vi "SP Initialize Test.vi"(0 "Instrument Record":T9, 2 "Files Found?":bool=TRUE, 5 "Parent VI Refnum":refnum<vi>, 7 "Timing Metrics In":string, 9 "Test Parameters":T10={"Stimulus"={"Use Instrument Settings"=FALSE, "Blank Frequencies"=FALSE, "Sweep Type"=enum."Linear", "Sweep"={"Fstart"=500.0, "Fstop"=1500.0, "Units"=enum."MHz", "Points"=2}, "Power (dBm)"=999.0, "IFBW (Hz)"=-1.0, "Sweep Time (s)"=-1.0, "Calibration"={"State"=FALSE, "String"=""}}, "Measurement"={"Auto Select"=TRUE, "Data Source"=enum."VNA", "Ports"=2, "Parameters"=[]}, "De-Embed"={"De-Embed"=FALSE, "Adapters"=[]}, "Display"={"Lock Control"=FALSE, "Retain Settings"=TRUE, "Formatted Data"=FALSE, "Plot Orientation"=enum."Single", "Plot Controls"=[{"Trace Orientation"=enum."Overlay", "Frequency"={"Change Frequency"=FALSE, "Start"=500.0, "Stop"=1500.0, "Units"=enum."MHz"}, "Markers"=[], "Traces"=[]}, {"Trace Orientation"=enum."Overlay", "Frequency"={"Change Frequency"=FALSE, "Start"=500.0, "Stop"=1500.0, "Units"=enum."MHz"}, "Markers"=[], "Traces"=[]}, {"Trace Orientation"=enum."Overlay", "Frequency"={"Change Frequency"=FALSE, "Start"=500.0, "Stop"=1500.0, "Units"=enum."MHz"}, "Markers"=[], "Traces"=[]}, {"Trace Orientation"=enum."Overlay", "Frequency"={"Change Frequency"=FALSE, "Start"=500.0, "Stop"=1500.0, "Units"=enum."MHz"}, "Markers"=[], "Traces"=[]}]}, "Limits"=[], "Filter Limits"=[]} {"Filter Limits"."Parameter"."Stimulus Port" min=1 step=1; "Filter Limits"."Parameter"."Response Port" min=1 step=1; "Filter Limits"."Passband"."Bandwidth Attn" format="%.3g"; "Filter Limits"."Passband"."Stop/Span" format="%.3g"; "Filter Limits"."Passband"."Start/Center" format="%.3g"; "Measurement"."Parameters"."Channel" min=0 max=32 step=1; "Measurement"."Parameters"."Parameter"."Stimulus Port" min=1 step=1; "Measurement"."Parameters"."Parameter"."Response Port" min=1 step=1; "Limits"."Parameter"."Stimulus Port" min=1 step=1; "Limits"."Parameter"."Response Port" min=1 step=1; "Stimulus"."Sweep Time (s)" format="%.3g"; "Display"."Plot Controls"."Traces"."Reference" format="%#.2g"; "Display"."Plot Controls"."Traces"."Display Data" items=["Data", "Memory", "Data/Memory"]; "Display"."Plot Controls"."Traces"."Format" items=["Log Mag", "Phase", "Expanded Phase", "Delay", "Smith", "Polar", "Lin Mag", "SWR", "Loss", "Real", "Imaginary"]; "Display"."Plot Controls"."Traces"."Scale" min=0.001 step=1.0 format="%#.2g"; "Display"."Plot Controls"."Traces"."Position" min=0.0 max=10.0; "Display"."Plot Controls"."Frequency"."Stop" format="%.3g"; "Display"."Plot Controls"."Frequency"."Start" format="%.3g"}, 11 "error in (no error)":errorcluster, 12 "Seq Count":u32) -> (4 "Instrument ID":string, 6 "Next Action":string, 8 "Timing Metrics Out":string, 10 "dup Test Parameters":T10={"Stimulus"={"Use Instrument Settings"=FALSE, "Blank Frequencies"=FALSE, "Sweep Type"=enum."Linear", "Sweep"={"Fstart"=500.0, "Fstop"=1500.0, "Units"=enum."MHz", "Points"=2}, "Power (dBm)"=999.0, "IFBW (Hz)"=-1.0, "Sweep Time (s)"=-1.0, "Calibration"={"State"=FALSE, "String"=""}}, "Measurement"={"Auto Select"=TRUE, "Data Source"=enum."VNA", "Ports"=2, "Parameters"=[]}, "De-Embed"={"De-Embed"=FALSE, "Adapters"=[]}, "Display"={"Lock Control"=FALSE, "Retain Settings"=TRUE, "Formatted Data"=FALSE, "Plot Orientation"=enum."Single", "Plot Controls"=[{"Trace Orientation"=enum."Overlay", "Frequency"={"Change Frequency"=FALSE, "Start"=500.0, "Stop"=1500.0, "Units"=enum."MHz"}, "Markers"=[], "Traces"=[]}, {"Trace Orientation"=enum."Overlay", "Frequency"={"Change Frequency"=FALSE, "Start"=500.0, "Stop"=1500.0, "Units"=enum."MHz"}, "Markers"=[], "Traces"=[]}, {"Trace Orientation"=enum."Overlay", "Frequency"={"Change Frequency"=FALSE, "Start"=500.0, "Stop"=1500.0, "Units"=enum."MHz"}, "Markers"=[], "Traces"=[]}, {"Trace Orientation"=enum."Overlay", "Frequency"={"Change Frequency"=FALSE, "Start"=500.0, "Stop"=1500.0, "Units"=enum."MHz"}, "Markers"=[], "Traces"=[]}]}, "Limits"=[], "Filter Limits"=[]} {"Filter Limits"."Parameter"."Stimulus Port" min=1 step=1; "Filter Limits"."Parameter"."Response Port" min=1 step=1; "Filter Limits"."Passband"."Bandwidth Attn" format="%.3g"; "Filter Limits"."Passband"."Stop/Span" format="%.3g"; "Filter Limits"."Passband"."Start/Center" format="%.3g"; "Measurement"."Parameters"."Channel" min=0 max=32 step=1; "Measurement"."Parameters"."Parameter"."Stimulus Port" min=1 step=1; "Measurement"."Parameters"."Parameter"."Response Port" min=1 step=1; "Limits"."Parameter"."Stimulus Port" min=1 step=1; "Limits"."Parameter"."Response Port" min=1 step=1; "Stimulus"."Sweep Time (s)" format="%.3g"; "Display"."Plot Controls"."Traces"."Reference" format="%#.2g"; "Display"."Plot Controls"."Traces"."Display Data" items=["Data", "Memory", "Data/Memory"]; "Display"."Plot Controls"."Traces"."Format" items=["Log Mag", "Phase", "Expanded Phase", "Delay", "Smith", "Polar", "Lin Mag", "SWR", "Loss", "Real", "Imaginary"]; "Display"."Plot Controls"."Traces"."Scale" min=0.001 step=1.0 format="%#.2g"; "Display"."Plot Controls"."Traces"."Position" min=0.0 max=10.0; "Display"."Plot Controls"."Frequency"."Stop" format="%.3g"; "Display"."Plot Controls"."Frequency"."Start" format="%.3g"}, 14 "Driver Ref":T5, 15 "error out":errorcluster {"code" format="%.0x"})   [LabVIEW 2011]
uses:
  TypeDefs/SP Test Parameters.ctl
  TypeDefs/SP Stimulus Parameters.ctl
  TypeDefs/SP Frequency Units.ctl
  TypeDefs/SP Calibration State.ctl
  TypeDefs/SP Measurement.ctl
  TypeDefs/SP Parameters.ctl
  TypeDefs/SP Parameter.ctl
  TypeDefs/SP De-Embed.ctl
  TypeDefs/SP Adapter.ctl
  TypeDefs/SP Data.ctl
  TypeDefs/SP Display Parameters.ctl
  TypeDefs/SP Display Plot Controls Cluster.ctl
  TypeDefs/SP Marker Cluster.ctl
  TypeDefs/SP Marker Type.ctl
  TypeDefs/SP Display Trace Controls.ctl
  TypeDefs/SP Display Format.ctl
  TypeDefs/SP Display Data.ctl
  TypeDefs/SP Limit.ctl
  TypeDefs/SP Format.ctl
  TypeDefs/SP Limit Type.ctl
  TypeDefs/SP Limit Point.ctl
  Test Referential Limit.ctl
  TypeDefs/SP Filter.ctl
  TypeDefs/SP Filter Type.ctl
  TypeDefs/SP Filter Passband.ctl
  TypeDefs/SP Frequency Format.ctl
  TypeDefs/SP Filter Ripple.ctl
  TypeDefs/SP Attenuation Point.ctl
  TypeDefs/SP Attenuation Type.ctl
  TypeDefs/SP Skirt Rejection Point.ctl
  TypeDefs/SP Relative Loss.ctl
  typedefs/Instrument Record.ctl
  TypeDefs/SP Driver Refs.ctl
  drivers/VNA/VNA Driver Ref.ctl
  drivers/SNA/SNA Driver Ref.ctl
  drivers/IMP/IMP Driver Ref.ctl
  TypeDefs/SP Parameter to Measure.ctl
  TypeDefs/SP Measurement Format.ctl
  TypeDefs/SP Miscellaneous Parameters.ctl
  drivers/VNA/VNA Command.ctl
  drivers/SNA/SNA Command.ctl
  drivers/IMP/IMP Command.ctl
panel:
  out "Parameters to Measure":T1[](array[typedef]) {"Channel" min=1 max=99 step=1; "Parameter"."Stimulus Port" min=1 step=1; "Parameter"."Response Port" min=1 step=1}
  # "Div"
  # "Div"
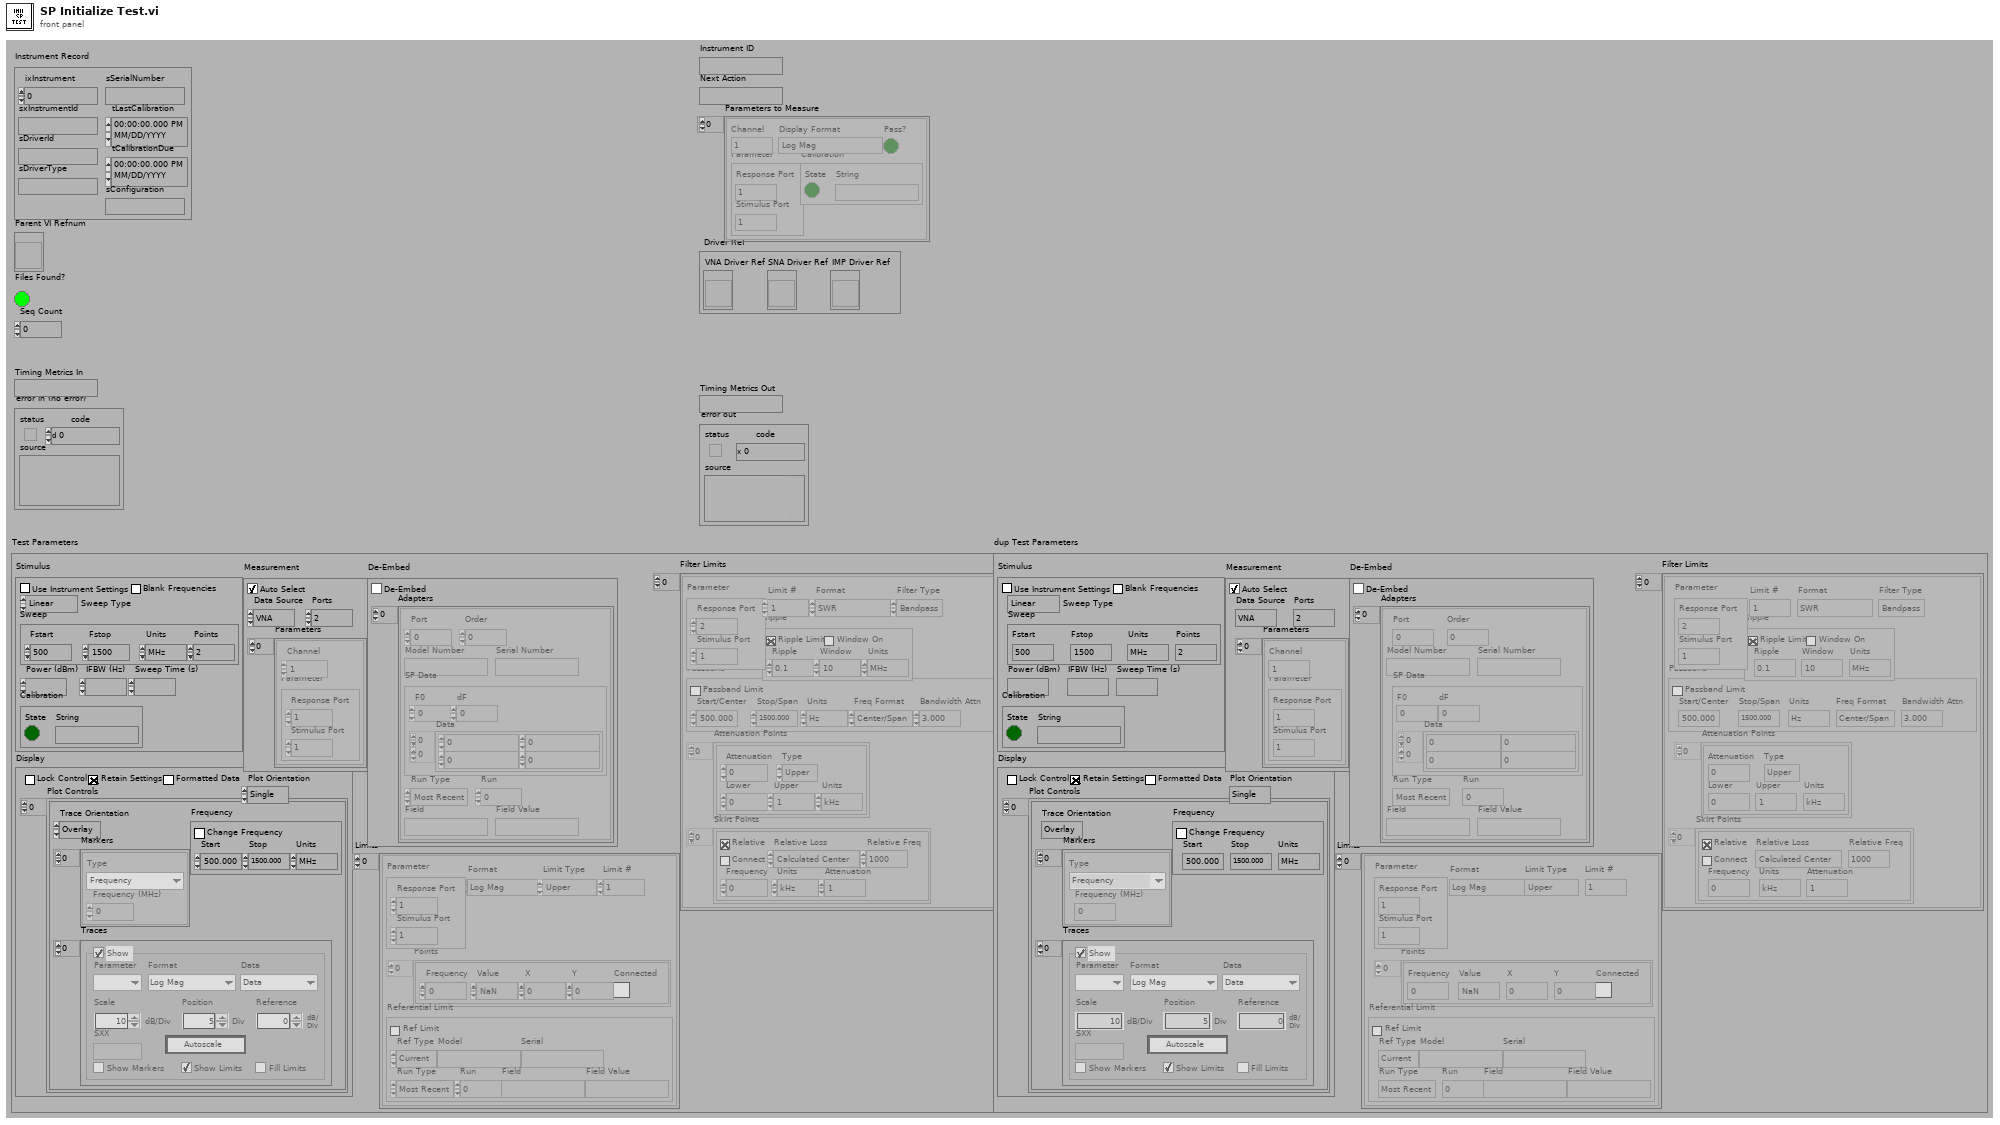
[diagram p1: front panel]
types:
  T1 = typedef "SP Parameter to Measure.ctl" = cluster{"Channel":i8, "Parameter":T2, "Calibration":T3, "Display Format":T4, "Pass?":bool}
  T2 = typedef "SP Parameter.ctl" = cluster{"Stimulus Port":i8, "Response Port":i8}
  T3 = typedef "SP Calibration State.ctl" = cluster{"State":bool, "String":string}
  T4 = typedef "SP Measurement Format.ctl" = enum32{"Log Mag", "Phase", "Delay", "Smith (R+jX)", "Polar (Re/Im)", "Linear Mag", "SWR", "Real", "Imaginary", "Smith (Lin/Phase)", "Smith (Log/Phase)", "Smith (Real/Imag)", "Smith (G+jB)", "Polar (Lin/Phase)", "Polar (Log/Phase)", "Expanded Phase", "Positive Phase", "Inverted Smith", "Unwrapped Phase", "Power Out", "Power In", "Linear Mag/Phase", "Log Mag/Phase", "Real/Imaginary"}
  T5 = typedef "SP Driver Refs.ctl" = cluster{"VNA Driver Ref":T6, "SNA Driver Ref":T7, "IMP Driver Ref":T8}
  T6 = typedef "VNA Driver Ref.ctl" = refnum<vi>
  T7 = typedef "SNA Driver Ref.ctl" = refnum<vi>
  T8 = typedef "IMP Driver Ref.ctl" = refnum<vi>
  T9 = typedef "Instrument Record.ctl" = cluster{"ixInstrument":i32, "sxInstrumentId":string, "sDriverId":string, "sDriverType":string, "sSerialNumber":string, "tLastCalibration":timestamp, "tCalibrationDue":timestamp, "sConfiguration":string}
  T10 = typedef "SP Test Parameters.ctl" = cluster{"Stimulus":T11, "Measurement":T13, "De-Embed":T15, "Display":T18, "Limits":T25[], "Filter Limits":T30[]}
  T11 = typedef "SP Stimulus Parameters.ctl" = cluster{"Use Instrument Settings":bool, "Blank Frequencies":bool, "Sweep Type":enum32{"Linear", "Logarithmic", "List", "Power", "CW"}, "Sweep":cluster{"Fstart":dbl, "Fstop":dbl, "Units":T12, "Points":i32}, "Power (dBm)":dbl, "IFBW (Hz)":dbl, "Sweep Time (s)":dbl, "Calibration":T3}
  T12 = typedef "SP Frequency Units.ctl" = enum16{"Hz", "kHz", "MHz", "GHz", "Points"}
  T13 = typedef "SP Measurement.ctl" = cluster{"Auto Select":bool, "Data Source":enum16{"VNA", "Data File"}, "Ports":i8, "Parameters":T14[]}
  T14 = typedef "SP Parameters.ctl" = cluster{"Channel":i8, "Parameter":T2}
  T15 = typedef "SP De-Embed.ctl" = cluster{"De-Embed":bool, "Adapters":T16[]}
  T16 = typedef "SP Adapter.ctl" = cluster{"Port":i8, "Order":i8, "Model Number":string, "Serial Number":string, "SP Data":T17, "Run Type":enum16{"Most Recent", "Run #", "Match Field"}, "Run":i32, "Field":string, "Field Value":string}
  T17 = typedef "SP Data.ctl" = cluster{"F0":dbl, "dF":dbl, "Data":cdb[][]}
  T18 = typedef "SP Display Parameters.ctl" = cluster{"Lock Control":bool, "Retain Settings":bool, "Formatted Data":bool, "Plot Orientation":enum32{"Single", "Dual", "Quad"}, "Plot Controls":T19[]}
  T19 = typedef "SP Display Plot Controls Cluster.ctl" = cluster{"Trace Orientation":enum32{"Overlay", "Split"}, "Frequency":cluster{"Change Frequency":bool, "Start":dbl, "Stop":dbl, "Units":T12}, "Markers":T20[], "Traces":T22[]}
  T20 = typedef "SP Marker Cluster.ctl" = cluster{"Type":T21, "Frequency (MHz)":dbl}
  T21 = typedef "SP Marker Type.ctl" = enum16{"Frequency", "Trace Maximum", "Trace Minimum", "Limit Maximum", "Limit Minimum"}
  T22 = typedef "SP Display Trace Controls.ctl" = cluster{"Trace On":bool, "Measure":i32, "Format":T23, "Autoscale":bool, "Reference":dbl, "\nRefUnit":string, "Position":dbl, "Scale":dbl, "ScaleUnit":string, "LimitOn":bool, "LimitFill":bool, "Display Data":T24, "Show Markers":bool, "SXX":string}
  T23 = typedef "SP Display Format.ctl" = i32
  T24 = typedef "SP Display Data.ctl" = u16
  T25 = typedef "SP Limit.ctl" = cluster{"Parameter":T2, "Format":T26, "Limit Type":T27, "Points":T28[], "Referential Limit":T29, "Limit #":i8}
  T26 = typedef "SP Format.ctl" = enum16{"Log Mag", "Lin Mag", "SWR", "Phase", "Expanded Phase", "Delay", "Insertion Loss", "Isolation", "Return Loss"}
  T27 = typedef "SP Limit Type.ctl" = enum16{"Upper", "Lower", "Delta", "Filter", "Referential"}
  T28 = typedef "SP Limit Point.ctl" = cluster{"Frequency":dbl, "Value":dbl, "X":dbl, "Y":dbl, "Connected":bool}
  T29 = typedef "Test Referential Limit.ctl" = cluster{"Ref Limit":bool, "Ref Type":enum16{"Current", "Specify"}, "Model":string, "Serial":string, "Run Type":enum16{"Most Recent", "Run #", "Match Field"}, "Run":i32, "Field":string, "Field Value":string}
  T30 = typedef "SP Filter.ctl" = cluster{"Limit #":i8, "Parameter":T2, "Format":T26, "Filter Type":T31, "Passband":T32, "Ripple":T34, "Attenuation Points":T35[], "Skirt Points":T37[]}
  T31 = typedef "SP Filter Type.ctl" = enum16{"Lowpass", "Highpass", "Bandpass", "Bandstop"}
  T32 = typedef "SP Filter Passband.ctl" = cluster{"Start/Center":dbl, "Stop/Span":dbl, "Units":T12, "Freq Format":T33, "Bandwidth Attn":dbl, "Passband Limit":bool}
  T33 = typedef "SP Frequency Format.ctl" = enum16{"Start/Stop", "Center/Span"}
  T34 = typedef "SP Filter Ripple.ctl" = cluster{"Ripple Limit":bool, "Window On":bool, "Ripple":dbl, "Window":dbl, "Units":T12}
  T35 = typedef "SP Attenuation Point.ctl" = cluster{"Attenuation":dbl, "Type":T36, "Lower":dbl, "Upper":dbl, "Units":T12}
  T36 = typedef "SP Attenuation Type.ctl" = enum16{"Center", "Lower", "Upper"}
  T37 = typedef "SP Skirt Rejection Point.ctl" = cluster{"Relative":bool, "Connect":bool, "Frequency":dbl, "Units":T12, "Attenuation":dbl, "Relative Loss":T38, "Relative Freq":dbl}
  T38 = typedef "SP Relative Loss.ctl" = enum16{"Calculated Center", "Passband Minimum", "Passband Maximum", "Passband Average", "Frequency"}
  T39 = typedef "SP Miscellaneous Parameters.ctl" = cluster{"Formatted Data":bool, "Auto Select":bool, "Seq Count":u32}
  T40 = typedef "VNA Command.ctl" = enum16{"LOAD", "INITIALIZE", "PRESET", "GET STIMULUS", "SET STIMULUS", "GET CALIBRATION", "CALIBRATE", "RESTORE", "MEASURE", "RELEASE", "UNLOAD", "CONFIRM", "SORT"}
  T41 = typedef "SNA Command.ctl" = enum16{"LOAD", "INITIALIZE", "PRESET", "GET STIMULUS", "SET STIMULUS", "GET CALIBRATION", "CALIBRATE", "RESTORE", "MEASURE", "RELEASE", "UNLOAD", "CONFIRM", "SORT"}
  T42 = enum16{"None", "Calibrate", "Restore", "Ignore", "Abort"}
  T43 = typedef "IMP Command.ctl" = enum16{"LOAD", "INITIALIZE", "IMPORT", "UNLOAD"}
  T44 = typedef "SP Dialog Response.ctl" = enum16{"None", "Calibrate", "Restore", "Ignore", "Abort", "Abort All"}
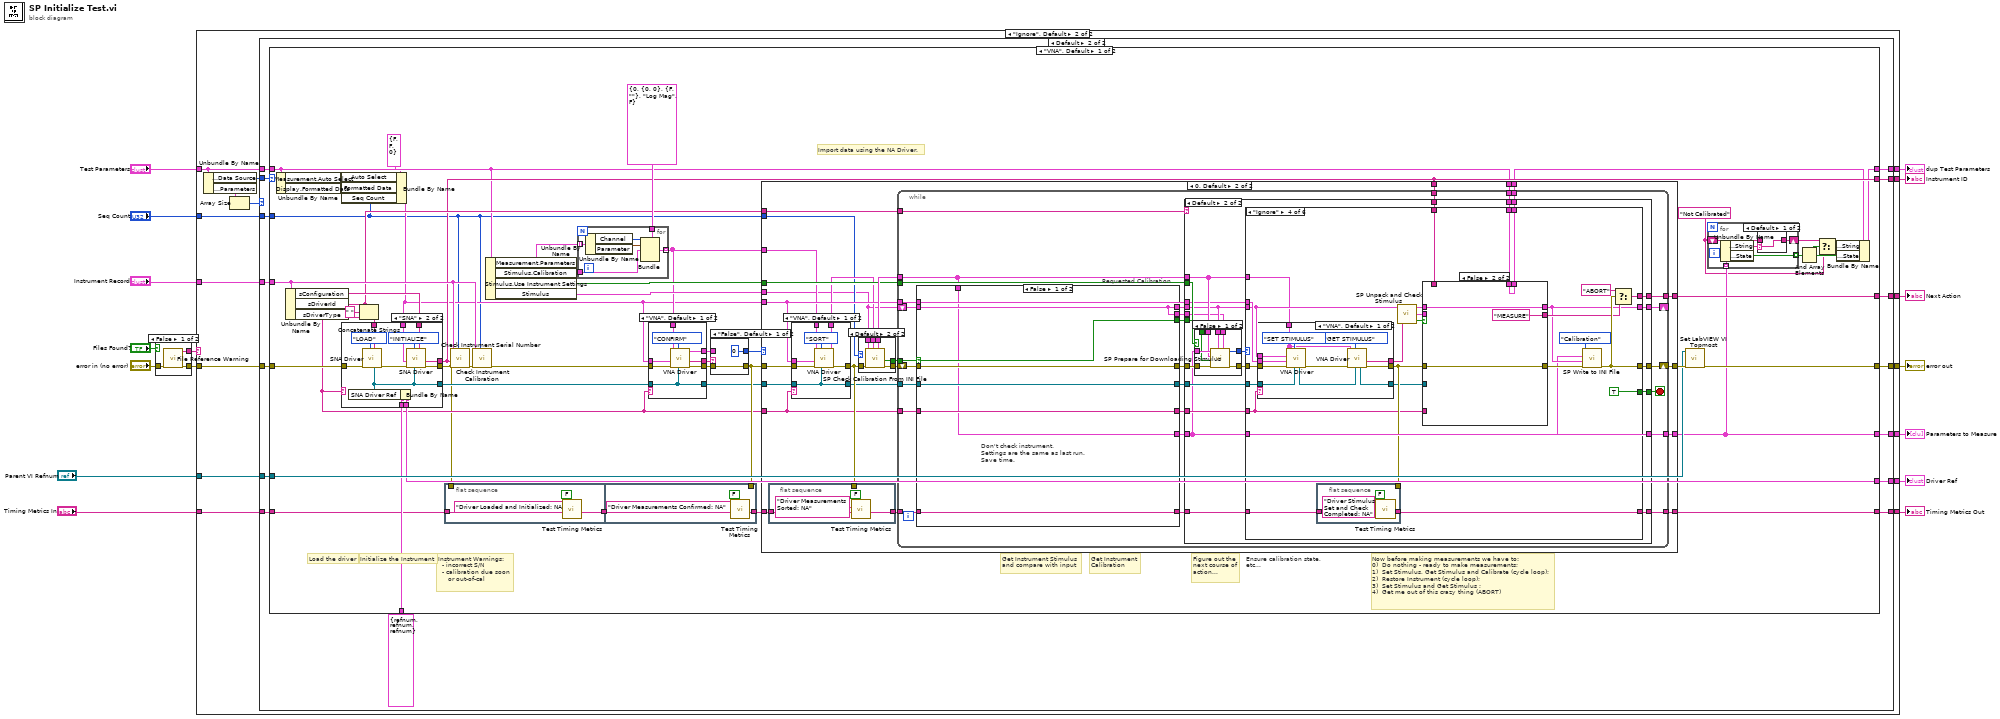
[diagram p0: block diagram]
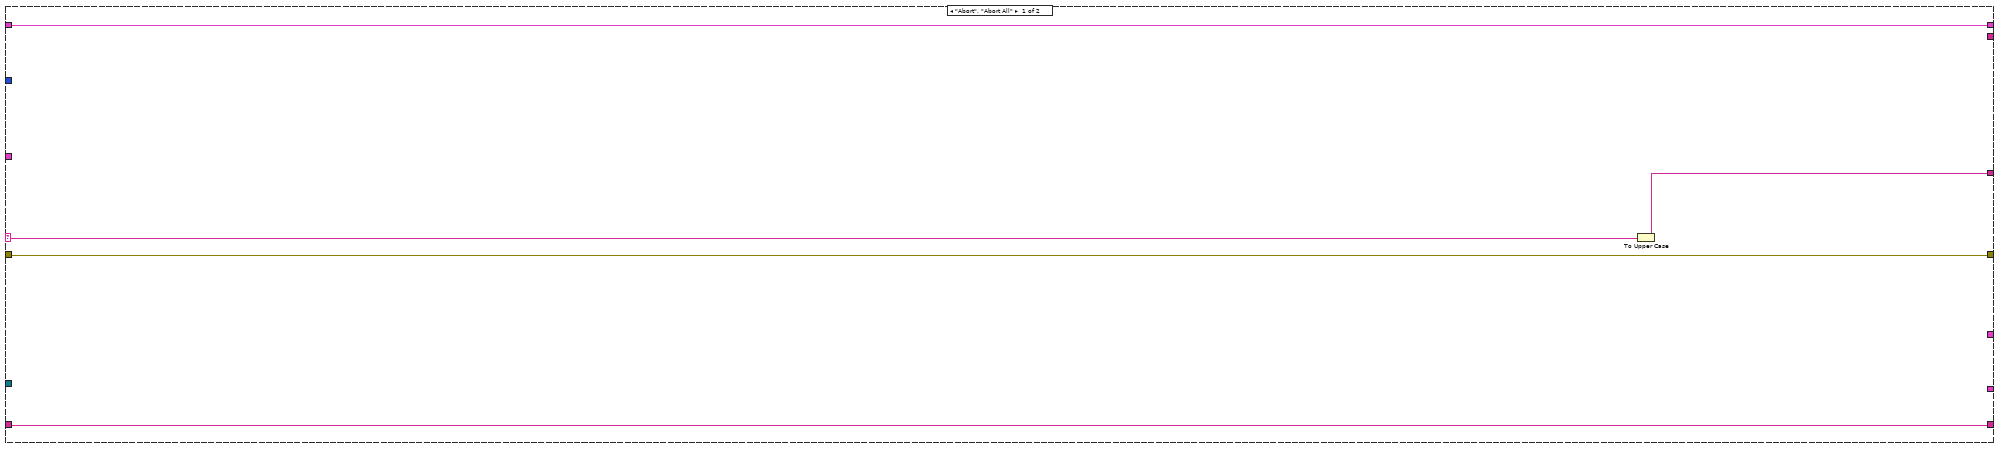
[diagram p3: hidden frame]
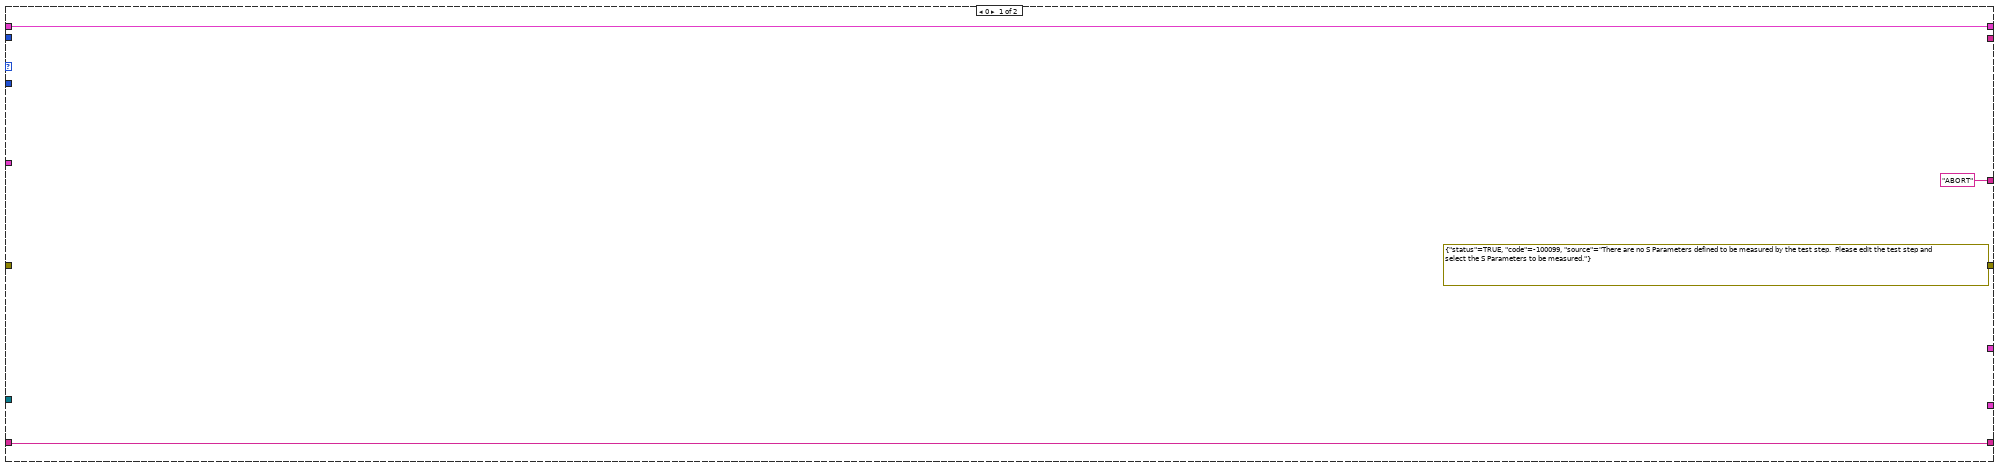
[diagram p4: hidden frame]
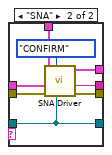
[diagram p6: hidden frame]
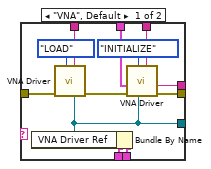
[diagram p7: hidden frame]
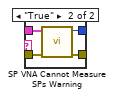
[diagram p8: hidden frame]
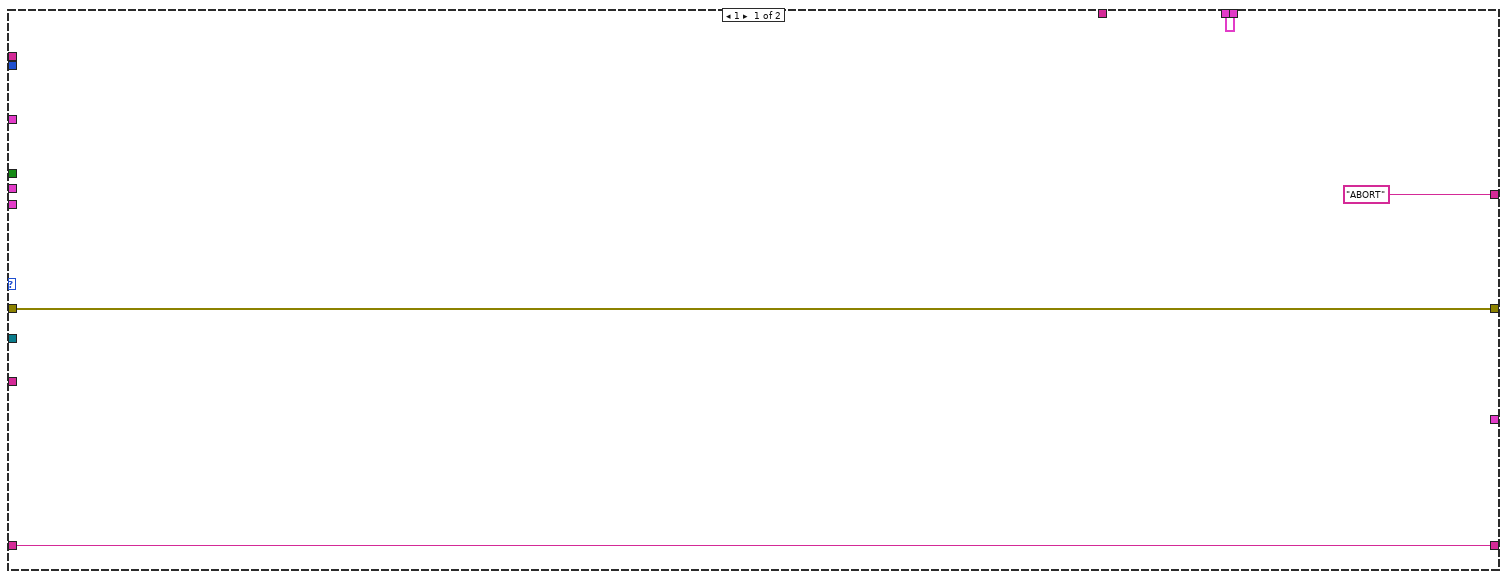
[diagram p9: hidden frame]
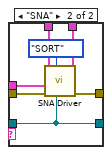
[diagram p10: hidden frame]
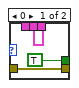
[diagram p11: hidden frame]
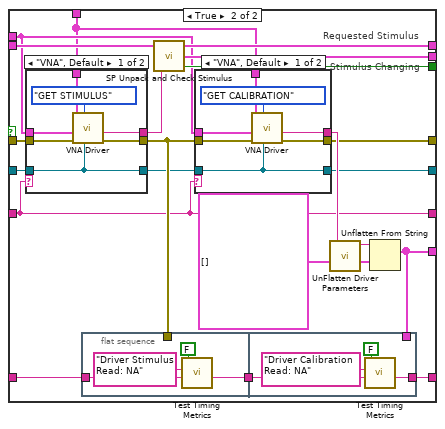
[diagram p12: hidden frame]
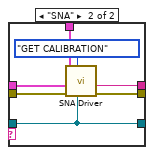
[diagram p13: hidden frame]
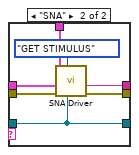
[diagram p14: hidden frame]
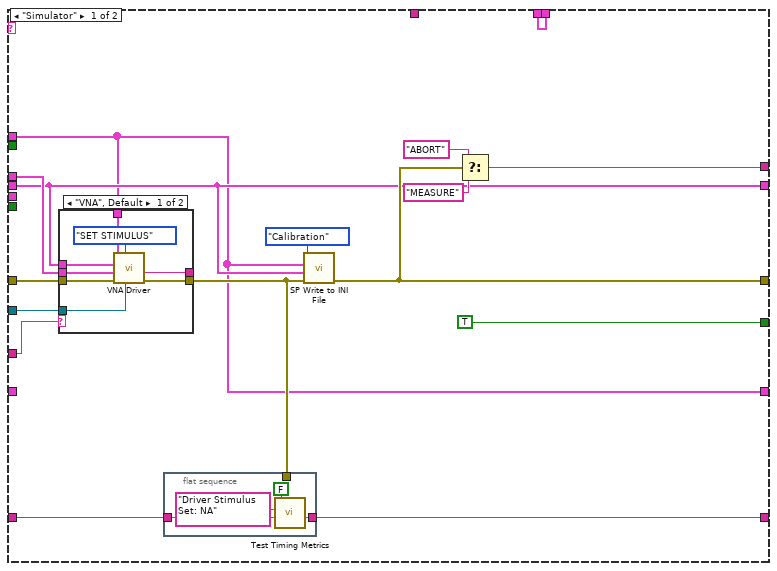
[diagram p15: hidden frame]
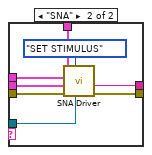
[diagram p16: hidden frame]
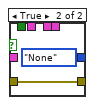
[diagram p17: hidden frame]
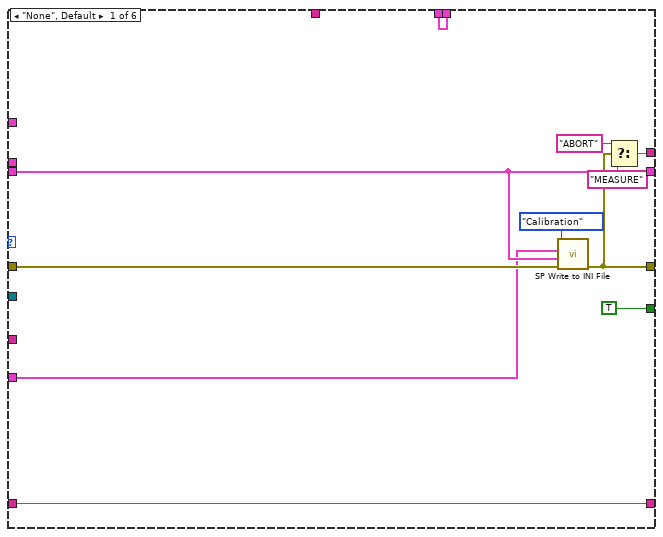
[diagram p18: hidden frame]
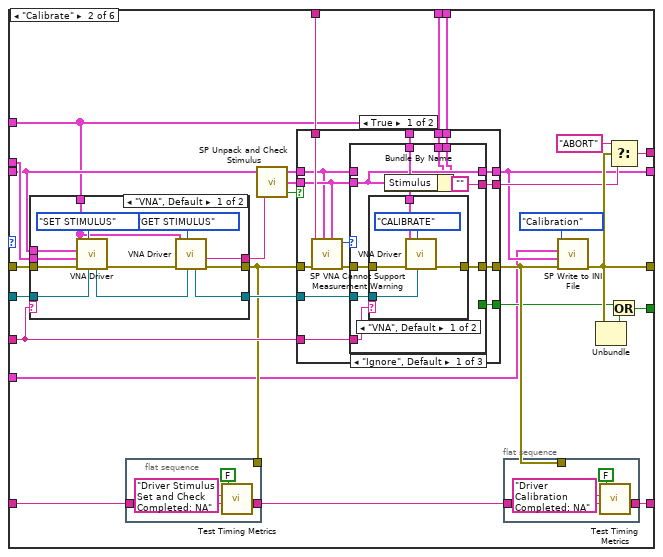
[diagram p19: hidden frame]
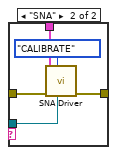
[diagram p20: hidden frame]
diagram:
  n1 = case shown="False" "Files Found?" {
    tunnel: "error in (no error)" -> [w19 w20]
    tunnel: [w18 w20] -> w4
    tunnel: [w17 _] -> w3
    frame False {
      n2 = call "File Reference Warning.vi"("error in (no error)"=w19) -> ("error out"=w18:errorcluster, "Command"=w17:string)  [unwired: 9 out]
    }
    frame True {
    }
  }
  n3 = case shown="\"Ignore\", Default" w3 {
    selector: w3 -> [w22 _]
    tunnel: w4 -> [w25 w41]
    tunnel: [_ w40] -> w16
    tunnel: "Instrument Record" -> [_ w39]
    tunnel: [w21 w38] -> w14
    tunnel: [_ w37] -> w13
    tunnel: [w25 w36] -> w12
    tunnel: "Parent VI Refnum" -> [_ w35]
    tunnel: "Test Parameters" -> [w23 w34]
    tunnel: [w23 w33] -> w9
    tunnel: [_ w32] -> w8
    tunnel: "Timing Metrics In" -> [w24 w30]
    tunnel: [w24 w29] -> w6
    tunnel: "Seq Count" -> [_ w28]
    frame "Abort", "Abort All" {
      n4 = To Upper Case(1:w22) -> (0:w21:string)
    }
    frame "Ignore", Default {
      n5 = Unbundle By Name(w34) -> ("Measurement.Data Source"=w31:enum16{"VNA", "Data File"}, "Measurement.Parameters"=w27:T14[])
      n6 = Array Size(array=w27) -> (size(s)=w26:i32)
      n7 = case shown="Default" w26 {
        tunnel: w41 -> [_ w60]
        tunnel: [_ w59] -> w40
        tunnel: w39 -> [_ w58]
        tunnel: ["ABORT" w57] -> w38
        tunnel: [_ w56] -> w37
        tunnel: [errorcluster {"status"=TRUE, "code"=-100099, "source"="There are no S Parameters defined to be measured by the test step.  Please edit the test step and select the S Parameters to be measured."} ("error out") w55] -> w36
        tunnel: w35 -> [_ w54]
        tunnel: w34 -> [w45 w53]
        tunnel: [w45 w52] -> w33
        tunnel: [_ w50] -> w32
        tunnel: w31 -> [_ w49]
        tunnel: w30 -> [w44 w48]
        tunnel: [w44 w47] -> w29
        tunnel: w28 -> [_ w46]
        frame 0 {
        }
        frame Default {
          n8 = case shown="\"VNA\", Default" w49 {
            tunnel: w60 -> [w108 w669]
            tunnel: [w77 w661] -> w59
            tunnel: w58 -> [w95 _]
            tunnel: [w106 "MEASURE"] -> w57
            tunnel: [w68 T1[] [{"Channel"=0, "Parameter"={"Stimulus Port"=0, "Response Port"=0}, "Calibration"={"State"=TRUE, "String"="Full 2-Port"}, "Display Format"=enum."Log Mag", "Pass?"=FALSE}] ("Parameters Measured")] -> w56
            tunnel: [w104 w660] -> w55
            tunnel: w54 -> [w103 _]
            tunnel: w53 -> [w74 w671]
            tunnel: [w66 w671] -> w52
            tunnel: T5 {"VNA Driver Ref"=refnum, "SNA Driver Ref"=refnum, "IMP Driver Ref"=refnum} ("Driver Ref") -> [w92 w667]
            tunnel: [w91 w666] -> w50
            tunnel: w48 -> [w75 w656]
            tunnel: [w81 w657] -> w47
            tunnel: w46 -> [w61 _]
            frame "VNA", Default {
              w62 = "Not Calibrated"
              # "Import data using the NA Driver."
              # "Now before making measurements we have to:\n0)  Do nothing - ready to make measurements;\n1)  Set Stimulus, Get Stimulus and Calibrate (cycle loop);\n2)  Restore Instrument (cycle loop);\n3)  Set Stimulus and Get Stimulus ;\n4)  Get me out of this crazy thing (ABORT)"
              # "Figure out the\nnext course of\naction..."
              # "Get Instrument\nCalibration"
              # "Instrument Warnings:\n  - incorrect S/N\n  - calibration due soon\n     or out-of-cal"
              # "Get Instrument Stimulus\nand compare with input"
              # "Initialize the Instrument"
              # "Load the driver"
              n9 = Unbundle By Name(w74) -> ("Measurement.Auto Select"=w72:bool, "Display.Formatted Data"=w71:bool)
              n10 = Unbundle By Name(w95) -> ("sConfiguration"=w94:string, "sDriverId"=w93:string, "sDriverType"=w80:string)
              n11 = Bundle By Name(cluster=T39 {"Formatted Data"=FALSE, "Auto Select"=FALSE, "Seq Count"=0} ("Miscellaneous Parameters"), "Auto Select"=w72, "Formatted Data"=w71, "Seq Count"=w61) -> (w70:T39)
              n12 = Concatenate Strings(w93, " " ("string"), w80) -> (w96:string)
              n13 = case shown="\"SNA\"" w80 {
                tunnel: w108 -> [w141 w153]
                tunnel: [w140 w152] -> w77
                tunnel: w96 -> [w139 w151]
                tunnel: w94 -> [w138 w150]
                tunnel: w92 -> [w137 w149]
                tunnel: [w136 w148] -> w91
                tunnel: [w134 w144] -> w79
                tunnel: [w133 w146] -> w76
                tunnel: w70 -> [w132 w145]
                frame "VNA", Default {
                  n14 = call "VNA Driver.vi"("VNA Driver or\nVNA Configuration (\"\")"=w139, "VNA Command"=VNA_Command."LOAD", "error in (no error)"=w141) -> ("error out"=w135:errorcluster, "dup Drv Refnum"=w134:T6)  [unwired: 4 in, 3 out]
                  n15 = Bundle By Name(cluster=w137, "VNA Driver Ref"=w134) -> (w136:T5)
                  n16 = call "VNA Driver.vi"("VNA Driver or\nVNA Configuration (\"\")"=w138, "Drv Refnum"=w134, "VNA Command"=VNA_Command."INITIALIZE", "error in (no error)"=w135, "Miscellaneous Parameters"=w132) -> ("error out"=w133:errorcluster, "VNA Flat Output"=w140:string)  [unwired: 2 in, 3 out]
                }
                frame "SNA" {
                  n17 = call "SNA Driver.vi"("SNA Driver or\nSNA Configuration (\"\")"=w151, "SNA Command"=SNA_Command."LOAD", "error in (no error)"=w153) -> ("error out"=w147:errorcluster, "dup Drv Refnum"=w144:T7)  [unwired: 4 in, 3 out]
                  n18 = Bundle By Name(cluster=w149, "SNA Driver Ref"=w144) -> (w148:T5)
                  n19 = call "SNA Driver.vi"("SNA Driver or\nSNA Configuration (\"\")"=w150, "Drv Refnum"=w144, "SNA Command"=SNA_Command."INITIALIZE", "error in (no error)"=w147, "Miscellaneous Parameters"=w145) -> ("error out"=w146:errorcluster, "SNA Flat Output"=w152:string)  [unwired: 2 in, 3 out]
                }
              }
              n20 = flat-sequence {
                tunnel: [w157] -> w85
                tunnel: w76 -> [_]
                tunnel: w75 -> [w156]
                tunnel: w85 -> [w161]
                tunnel: w83 -> [_]
                tunnel: [w160] -> w82
                frame #0 {
                  n21 = call "Test Timing Metrics.vi"("Start?"=FALSE, "Timing Metrics In"=w156, "Message"="Driver Loaded and Initialized: NA") -> ("Timing Metrics Out"=w157:string)  [unwired: 6 out]
                }
                frame #1 {
                  n22 = call "Test Timing Metrics.vi"("Start?"=FALSE, "Timing Metrics In"=w161, "Message"="Driver Measurements Confirmed: NA") -> ("Timing Metrics Out"=w160:string)  [unwired: 6 out]
                }
              }
              n23 = call "Check Instrument Serial Number.vi"("Seq Count"=w61, "error in (no error)"=w76, "Instrument IDN String (\"\")"=w77, "Instrument Record"=w95) -> ("error out"=w107:errorcluster)  [unwired: 7 out]
              n24 = call "Check Instrument Calibration.vi"("Seq Count"=w61, "error in (no error)"=w107, "Instrument Record"=w95) -> ("error out"=w90:errorcluster)  [unwired: 8 out]
              n25 = Unbundle By Name(w74) -> ("Measurement.Parameters"=w102:T14[], "Stimulus.Calibration"=w100:T3, "Stimulus.Use Instrument Settings"=w98:bool, "Stimulus"=w99:T11)
              n26 = for {
                tunnel: [w169] -> w86 mode=indexing
                tunnel: T1 {"Channel"=0, "Parameter"={"Stimulus Port"=0, "Response Port"=0}, "Calibration"={"State"=FALSE, "String"=""}, "Display Format"=enum."Log Mag", "Pass?"=FALSE} ("Parameter to Measure") -> [w168]
                tunnel: w100 -> [w167]
                tunnel: w102 -> [w166] mode=indexing
                n27 = Unbundle By Name(w166) -> ("Channel"=w164:i8, "Parameter"=w165:T2)
                n28 = Bundle(cluster=w168, "Channel"=w164, "Parameter"=w165, "Calibration"=w167) -> (w169:T1)  [unwired: 2 out]
              }
              n29 = case shown="\"VNA\", Default" w80 {
                tunnel: w90 -> [w122 w130]
                tunnel: w70 -> [w121 w129]
                tunnel: [w120 w128] -> w89
                tunnel: [w119 w127] -> w88
                tunnel: w86 -> [w118 w126]
                tunnel: [w117 w125] -> w84
                tunnel: w79 -> [w116 w124]
                tunnel: [w116 w124] -> w78
                frame "VNA", Default {
                  n30 = call "VNA Driver.vi"("Drv Refnum"=w116, "VNA Command"=VNA_Command."CONFIRM", "error in (no error)"=w122, "Miscellaneous Parameters"=w121, "Parameters to Measure"=w118) -> ("error out"=w117:errorcluster, "VNA Flat Output"=w120:string, "Parameters Measured"=w119:T1[])  [unwired: 2 in, 2 out]
                }
                frame "SNA" {
                  n31 = call "SNA Driver.vi"("Drv Refnum"=w124, "SNA Command"=SNA_Command."CONFIRM", "error in (no error)"=w130, "Miscellaneous Parameters"=w129, "Parameters to Measure"=w126) -> ("error out"=w125:errorcluster, "SNA Flat Output"=w128:string, "Parameters Measured"=w127:T1[])  [unwired: 2 in, 2 out]
                }
              }
              n32 = case shown="\"False\", Default" w89 {
                tunnel: w84 -> [w171 w175]
                tunnel: [w171 w174] -> w83
                tunnel: w88 -> [_ w173]
                tunnel: [0 ("Choice") w172] -> w87
                frame "False", Default {
                }
                frame "True" {
                  n33 = call "SP VNA Cannot Measure SPs Warning.vi"("error in (no error)"=w175, "Removed Parameters"=w173) -> ("error out"=w174:errorcluster, "Choice"=w172:i32)  [unwired: 8 out]
                }
              }
              n34 = case shown="0, Default" w87 {
                tunnel: ["ABORT" w203] -> w106
                tunnel: [_ w200] -> w68
                tunnel: [w179 w199] -> w105
                tunnel: w99 -> [_ w180]
                tunnel: w98 -> [_ w197]
                tunnel: w93 -> [_ w196]
                tunnel: w83 -> [w179 w191]
                tunnel: w70 -> [_ w190]
                tunnel: w86 -> [_ w189]
                tunnel: w82 -> [w177 w195]
                tunnel: [w177 w193] -> w81
                tunnel: w80 -> [_ w185]
                tunnel: w78 -> [_ w187]
                tunnel: w77 -> [_ w184]
                tunnel: w74 -> [w176 w183]
                tunnel: [w176 w182] -> w67
                tunnel: w61 -> [_ w181]
                frame 1 {
                }
                frame 0, Default {
                  n35 = flat-sequence {
                    tunnel: w195 -> [w219]
                    tunnel: [w218] -> w194
                    tunnel: w192 -> [_]
                    frame #0 {
                      n36 = call "Test Timing Metrics.vi"("Start?"=FALSE, "Timing Metrics In"=w219, "Message"="Driver Measurements Sorted: NA") -> ("Timing Metrics Out"=w218:string)  [unwired: 6 out]
                    }
                  }
                  n37 = case shown="\"VNA\", Default" w185 {
                    tunnel: w191 -> [w209 w216]
                    tunnel: w190 -> [w208 w215]
                    tunnel: w189 -> [w207 w214]
                    tunnel: [w206 w213] -> w192
                    tunnel: [w205 w212] -> w188
                    tunnel: w187 -> [w204 w211]
                    tunnel: [w204 w211] -> w186
                    frame "VNA", Default {
                      n38 = call "VNA Driver.vi"("Drv Refnum"=w204, "VNA Command"=VNA_Command."SORT", "error in (no error)"=w209, "Miscellaneous Parameters"=w208, "Parameters to Measure"=w207) -> ("error out"=w206:errorcluster, "Parameters Measured"=w205:T1[])  [unwired: 2 in, 3 out]
                    }
                    frame "SNA" {
                      n39 = call "SNA Driver.vi"("Drv Refnum"=w211, "SNA Command"=SNA_Command."SORT", "error in (no error)"=w216, "Miscellaneous Parameters"=w215, "Parameters to Measure"=w214) -> ("error out"=w213:errorcluster, "Parameters Measured"=w212:T1[])  [unwired: 2 in, 3 out]
                    }
                  }
                  n40 = case shown="Default" w181 {
                    tunnel: w192 -> [w224 w230]
                    tunnel: [w224 w229] -> w202
                    tunnel: [TRUE ("Check Instrument") w228] -> w201
                    tunnel: w188 -> [w222 w227]
                    tunnel: w180 -> [_ w226]
                    tunnel: [w222 w225] -> w198
                    frame 0 {
                    }
                    frame Default {
                      n41 = call "SP Check Calibration From INI File.vi"("Paramters to Measure"=w227, "error in (no error)"=w230, "Requested Stimulus"=w226) -> ("error out"=w229:errorcluster, "Check Instrument"=w228:bool, "Paramters to Measure Out"=w225:T1[])  [unwired: 6 out]
                    }
                  }
                  n42 = while "Ensure calibration state, etc..." {
                    shift-right: [w256] -> w199
                    shift-left: w202 -> [w245]
                    tunnel: [w255] -> w203
                    tunnel: [w253] -> w200
                    tunnel: w196 -> [w252]
                    tunnel: w198 -> [w231]
                    tunnel: w201 -> [w246]
                    tunnel: w197 -> [w244]
                    tunnel: w190 -> [w242]
                    tunnel: w194 -> [w241]
                    tunnel: [w239] -> w193
                    tunnel: w186 -> [w238]
                    tunnel: w185 -> [w237]
                    tunnel: w184 -> [w235]
                    tunnel: w183 -> [w234]
                    tunnel: [w233] -> w182
                    shift-right: [w232] -> _
                    shift-left: w180 -> [w247]
                    stop <- w257 stop-if-true
                    # "Requested Calibration"
                    n43 = case shown="False" w246 {
                      selector: w246 -> [w263 _]
                      tunnel: [w258 w278] -> w254
                      tunnel: [w264 w272] -> w251
                      tunnel: [w263 w283] -> w250
                      tunnel: [w262 w284] -> w249
                      tunnel: w245 -> [w264 w276]
                      tunnel: w247 -> [w262 w282]
                      tunnel: [w260 w268] -> w248
                      tunnel: [w262 w281] -> w243
                      tunnel: w231 -> [w258 w267]
                      tunnel: w242 -> [_ w271]
                      tunnel: w241 -> [w261 w280]
                      tunnel: [w261 w277] -> w240
                      tunnel: w238 -> [w260 w275]
                      tunnel: w237 -> [w259 w266]
                      tunnel: [w259 w266] -> w236
                      frame False {
                        # "Don't check instrument.\nSettings are the same as last run.\nSave time."
                      }
                      frame True {
                        # "Requested Stimulus"
                        # "Stimulus Changing"
                        n44 = case shown="\"VNA\", Default" w266 {
                          tunnel: w276 -> [w306 w313]
                          tunnel: w271 -> [w305 w312]
                          tunnel: w267 -> [w304 w311]
                          tunnel: [w303 w310] -> w270
                          tunnel: w275 -> [w302 w309]
                          tunnel: [w302 w309] -> w269
                          tunnel: [w301 w308] -> w274
                          frame "VNA", Default {
                            n45 = call "VNA Driver.vi"("Drv Refnum"=w302, "VNA Command"=VNA_Command."GET STIMULUS", "error in (no error)"=w306, "Miscellaneous Parameters"=w305, "Parameters to Measure"=w304) -> ("error out"=w303:errorcluster, "VNA Flat Output"=w301:string)  [unwired: 2 in, 3 out]
                          }
                          frame "SNA" {
                            n46 = call "SNA Driver.vi"("Drv Refnum"=w309, "SNA Command"=SNA_Command."GET STIMULUS", "error in (no error)"=w313, "Miscellaneous Parameters"=w312, "Parameters to Measure"=w311) -> ("error out"=w310:errorcluster, "SNA Flat Output"=w308:string)  [unwired: 2 in, 3 out]
                          }
                        }
                        n47 = flat-sequence {
                          tunnel: w280 -> [w315]
                          tunnel: w270 -> [_]
                          tunnel: [w314] -> w279
                          tunnel: w279 -> [w319]
                          tunnel: w278 -> [_]
                          tunnel: [w318] -> w277
                          frame #0 {
                            n48 = call "Test Timing Metrics.vi"("Start?"=FALSE, "Timing Metrics In"=w315, "Message"="Driver Stimulus Read: NA") -> ("Timing Metrics Out"=w314:string)  [unwired: 6 out]
                          }
                          frame #1 {
                            n49 = call "Test Timing Metrics.vi"("Start?"=FALSE, "Timing Metrics In"=w319, "Message"="Driver Calibration Read: NA") -> ("Timing Metrics Out"=w318:string)  [unwired: 6 out]
                          }
                        }
                        n50 = call "SP Unpack and Check Stimulus.vi"("Flat Stimulus"=w274, "Requested Stimulus In"=w282) -> ("Stimulus Changed?"=w283:bool, "Current Stimulus"=w281:T11, "Requested Stimulus Out"=w284:T11)  [unwired: 1 out]
                        n51 = case shown="\"VNA\", Default" w266 {
                          tunnel: w270 -> [w292 w299]
                          tunnel: w271 -> [w291 w298]
                          tunnel: w267 -> [w290 w297]
                          tunnel: [w289 w296] -> w272
                          tunnel: w269 -> [w288 w295]
                          tunnel: [w288 w295] -> w268
                          tunnel: [w287 w294] -> w273
                          frame "VNA", Default {
                            n52 = call "VNA Driver.vi"("Drv Refnum"=w288, "VNA Command"=VNA_Command."GET CALIBRATION", "error in (no error)"=w292, "Miscellaneous Parameters"=w291, "Parameters to Measure"=w290) -> ("error out"=w289:errorcluster, "VNA Flat Output"=w287:string)  [unwired: 2 in, 3 out]
                          }
                          frame "SNA" {
                            n53 = call "SNA Driver.vi"("Drv Refnum"=w295, "SNA Command"=SNA_Command."GET CALIBRATION", "error in (no error)"=w299, "Miscellaneous Parameters"=w298, "Parameters to Measure"=w297) -> ("error out"=w296:errorcluster, "SNA Flat Output"=w294:string)  [unwired: 2 in, 3 out]
                          }
                        }
                        n54 = call "UnFlatten Driver Parameters.vi"("Flattened Driver Parameters with Version (\"\")"=w273) -> ("Flat Driver Parameters"=w285:string)  [unwired: 1 in, 5 out]
                        n55 = Unflatten From String(type=T1[] [] ("Parameters Measured"), binary string=w285) -> (value=w278:T1[])  [unwired: 1 in, 4 out]
                      }
                    }
                    n56 = case shown="Default" w252 {
                      tunnel: [TRUE w378] -> w257
                      tunnel: [w333 w377] -> w256
                      tunnel: [w335 w376] -> w255
                      tunnel: w249 -> [w323 w369]
                      tunnel: w248 -> [w326 w375]
                      tunnel: w254 -> [_ w358]
                      tunnel: [w322 w358] -> w253
                      tunnel: w251 -> [w328 w374]
                      tunnel: w231 -> [w322 w371]
                      tunnel: w250 -> [_ w363]
                      tunnel: w244 -> [_ w370]
                      tunnel: w243 -> [_ w368]
                      tunnel: w242 -> [w329 w367]
                      tunnel: w240 -> [w330 w366]
                      tunnel: [w331 w365] -> w239
                      tunnel: w236 -> [w325 w364]
                      tunnel: w235 -> [_ w362]
                      tunnel: w234 -> [w324 w361]
                      tunnel: [w324 w360] -> w233
                      tunnel: [w323 w359] -> w232
                      frame "Simulator" {
                        n57 = case shown="\"VNA\", Default" w325 {
                          tunnel: w328 -> [w345 w353]
                          tunnel: w329 -> [w344 w352]
                          tunnel: w322 -> [w343 w351]
                          tunnel: [w342 w350] -> w327
                          tunnel: w326 -> [w341 w349]
                          tunnel: [w340 w348] -> _
                          tunnel: w323 -> [w338 w346]
                          frame "VNA", Default {
                            n58 = call "VNA Driver.vi"("Drv Refnum"=w341, "VNA Command"=VNA_Command."SET STIMULUS", "error in (no error)"=w345, "Miscellaneous Parameters"=w344, "VNA Stimulus"=w338, "Parameters to Measure"=w343) -> ("error out"=w342:errorcluster, "VNA Flat Output"=w340:string)  [unwired: 1 in, 3 out]
                          }
                          frame "SNA" {
                            n59 = call "SNA Driver.vi"("Drv Refnum"=w349, "SNA Command"=SNA_Command."SET STIMULUS", "error in (no error)"=w353, "Miscellaneous Parameters"=w352, "SNA Stimulus"=w346, "Parameters to Measure"=w351) -> ("error out"=w350:errorcluster, "SNA Flat Output"=w348:string)  [unwired: 1 in, 3 out]
                          }
                        }
                        n60 = flat-sequence {
                          tunnel: [w354] -> w331
                          tunnel: w330 -> [w355]
                          tunnel: w327 -> [_]
                          frame #0 {
                            n61 = call "Test Timing Metrics.vi"("Start?"=FALSE, "Timing Metrics In"=w355, "Message"="Driver Stimulus Set: NA") -> ("Timing Metrics Out"=w354:string)  [unwired: 6 out]
                          }
                        }
                        n62 = call "SP Write to INI File.vi"("error in (no error)"=w327, "Requested Stimulus"=w323, "Parameters to Measure"=w322, "Data to Write"=enum16{"Calibration", "Display", "De-Embed"}."Calibration") -> ("error out"=w333:errorcluster)  [unwired: 3 in, 4 out]
                        n63 = Select(t="ABORT", s=w333, f="MEASURE") -> (s? t:f=w335:string)
                      }
                      frame Default {
                        n64 = case shown="False" w370 {
                          tunnel: w374 -> [w386 w388]
                          tunnel: [w385 w388] -> w373
                          tunnel: [w384 T42."None" ("Action")] -> w372
                          tunnel: w358 -> [w383 _]
                          tunnel: w363 -> [w382 _]
                          tunnel: w371 -> [w381 _]
                          tunnel: w369 -> [w380 _]
                          tunnel: w368 -> [w379 _]
                          frame False {
                            n65 = call "SP Prepare for Downloading Stimulus.vi"("Current Stimulus"=w379, "Requested Stimulus"=w380, "error in (no error)"=w386, "Stimulus Changing? (f)"=w382, "Parameters to Measure"=w381, "Currnet Parameters to Measure"=w383) -> ("error out"=w385:errorcluster, "Action"=w384:T44)  [unwired: 1 in, 3 out]
                          }
                          frame True {
                          }
                        }
                        n66 = case shown="\"Ignore\"" w372 {
                          tunnel: w373 -> [w395 w423 w530 w563 w642 w650]
                          tunnel: [w394 w426 w534 w574 w641 w649] -> w377
                          tunnel: [TRUE w407 w535 TRUE TRUE TRUE] -> w378
                          tunnel: [w397 w427 w536 w578 "ABORT" "ABORT ALL"] -> w376
                          tunnel: w375 -> [_ w422 w528 w571 _ _]
                          tunnel: w371 -> [_ w400 w523 w553 _ _]
                          tunnel: w369 -> [w390 w417 w525 w561 w638 w646]
                          tunnel: w367 -> [_ w421 _ w562 _ _]
                          tunnel: w366 -> [w392 w415 w532 w570 w640 w648]
                          tunnel: [w392 w424 w531 w569 w640 w648] -> w365
                          tunnel: w364 -> [_ w418 w527 w564 _ _]
                          tunnel: w362 -> [_ w412 _ w559 _ _]
                          tunnel: w361 -> [w391 w404 w526 w557 w639 w647]
                          tunnel: [w391 w403 w526 w556 w639 w647] -> w360
                          tunnel: [w390 w402 w525 w555 w638 w646] -> w359
                          tunnel: w358 -> [w389 w401 w524 w554 w637 w645]
                          frame "None", Default {
                            n67 = call "SP Write to INI File.vi"("error in (no error)"=w395, "Requested Stimulus"=w390, "Parameters to Measure"=w389, "Data to Write"=enum16{"Calibration", "Display", "De-Embed"}."Calibration") -> ("error out"=w394:errorcluster)  [unwired: 3 in, 4 out]
                            n68 = Select(t="ABORT", s=w394, f="MEASURE") -> (s? t:f=w397:string)
                          }
                          frame "Calibrate" {
                            n69 = case shown="\"VNA\", Default" w418 {
                              tunnel: w423 -> [w506 w518]
                              tunnel: w421 -> [w505 w508]
                              tunnel: w400 -> [w497 w512]
                              tunnel: [w500 w513] -> w413
                              tunnel: w422 -> [w502 w511]
                              tunnel: w417 -> [w503 w516]
                              tunnel: [w496 w509] -> w419
                              tunnel: [w495 w507] -> w416
                              frame "VNA", Default {
                                n70 = call "VNA Driver.vi"("Drv Refnum"=w502, "VNA Command"=VNA_Command."SET STIMULUS", "error in (no error)"=w506, "Miscellaneous Parameters"=w505, "VNA Stimulus"=w503, "Parameters to Measure"=w497) -> ("error out"=w498:errorcluster, "dup Drv Refnum"=w501:T6)  [unwired: 1 in, 3 out]
                                n71 = call "VNA Driver.vi"("Drv Refnum"=w501, "VNA Command"=VNA_Command."GET STIMULUS", "error in (no error)"=w498, "Parameters to Measure"=w497) -> ("error out"=w500:errorcluster, "VNA Flat Output"=w495:string, "dup Drv Refnum"=w496:T6)  [unwired: 3 in, 2 out]
                              }
                              frame "SNA" {
                                n72 = call "SNA Driver.vi"("Drv Refnum"=w511, "SNA Command"=SNA_Command."SET STIMULUS", "error in (no error)"=w518, "Miscellaneous Parameters"=w508, "SNA Stimulus"=w516, "Parameters to Measure"=w512) -> ("error out"=w514:errorcluster, "dup Drv Refnum"=w510:T7)  [unwired: 1 in, 3 out]
                                n73 = call "SNA Driver.vi"("Drv Refnum"=w510, "SNA Command"=SNA_Command."GET STIMULUS", "error in (no error)"=w514, "Miscellaneous Parameters"=w508, "Parameters to Measure"=w512) -> ("error out"=w513:errorcluster, "SNA Flat Output"=w507:string, "dup Drv Refnum"=w509:T7)  [unwired: 2 in, 2 out]
                              }
                            }
                            n74 = flat-sequence {
                              tunnel: [w492] -> w414
                              tunnel: w415 -> [w491]
                              tunnel: w413 -> [_]
                              frame #0 {
                                n75 = call "Test Timing Metrics.vi"("Start?"=FALSE, "Timing Metrics In"=w491, "Message"="Driver Stimulus Set and Check Completed: NA") -> ("Timing Metrics Out"=w492:string)  [unwired: 6 out]
                              }
                            }
                            n76 = call "SP Unpack and Check Stimulus.vi"("Flat Stimulus"=w416, "Requested Stimulus In"=w417) -> ("Stimulus Changed?"=w411:bool, "Current Stimulus"=w410:T11, "Requested Stimulus Out"=w409:T11)  [unwired: 1 out]
                            n77 = case shown="True" w411 {
                              tunnel: [w443 w480] -> w420
                              tunnel: w419 -> [w442 w479]
                              tunnel: w400 -> [w441 w478]
                              tunnel: w418 -> [w440 w477]
                              tunnel: w413 -> [w438 w475]
                              tunnel: w412 -> [w437 _]
                              tunnel: w410 -> [w435 _]
                              tunnel: w409 -> [w434 w474]
                              tunnel: [w433 w474] -> w402
                              tunnel: [w432 ""] -> w408
                              tunnel: [w431 _] -> w405
                              tunnel: w404 -> [w430 w473]
                              tunnel: [w429 w473] -> w403
                              frame True {
                                n78 = call "SP VNA Cannot Support Measurement Warning.vi"("Current Stimulus"=w435, "Requested Stimulus"=w434, "error in (no error)"=w438, "Instrument IDN String (\"\")"=w437) -> ("error out"=w439:errorcluster, "Choice"=w436:T44)  [unwired: 2 in, 4 out]
                                n79 = case shown="\"Ignore\", Default" w436 {
                                tunnel: [w452 w465 w470] -> w443
                                tunnel: w442 -> [w451 _ _]
                                tunnel: w441 -> [w450 _ _]
                                tunnel: w440 -> [w449 _ _]
                                tunnel: w439 -> [w448 w465 w470]
                                tunnel: w435 -> [w446 _ _]
                                tunnel: w434 -> [_ w467 w472]
                                tunnel: [w446 w467 w472] -> w433
                                tunnel: ["" "ABORT" "ABORT ALL"] -> w432
                                tunnel: [_ TRUE TRUE] -> w431
                                tunnel: w430 -> [w445 w463 w468]
                                tunnel: [w444 w463 w468] -> w429
                                frame "Ignore", Default {
                                n80 = case shown="\"VNA\", Default" w449 {
                                tunnel: w448 -> [w457 w462]
                                tunnel: w450 -> [w454 w460]
                                tunnel: [w453 w458] -> w452
                                tunnel: w451 -> [w455 w459]
                                frame "VNA", Default {
                                n81 = call "VNA Driver.vi"("Drv Refnum"=w455, "VNA Command"=VNA_Command."CALIBRATE", "error in (no error)"=w457, "Parameters to Measure"=w454) -> ("error out"=w453:errorcluster)  [unwired: 3 in, 4 out]
                                }
                                frame "SNA" {
                                n82 = call "SNA Driver.vi"("Drv Refnum"=w459, "SNA Command"=SNA_Command."CALIBRATE", "error in (no error)"=w462, "Parameters to Measure"=w460) -> ("error out"=w458:errorcluster)  [unwired: 3 in, 4 out]
                                }
                                }
                                n83 = Bundle By Name(cluster=w445, "Stimulus"=w446) -> (w444:T10)
                                }
                                frame "Abort" {
                                }
                                frame "Abort All" {
                                }
                                }
                              }
                              frame False {
                                n84 = case shown="\"VNA\", Default" w477 {
                                tunnel: w475 -> [w485 w490]
                                tunnel: w478 -> [w482 w488]
                                tunnel: [w481 w486] -> w480
                                tunnel: w479 -> [w483 w487]
                                frame "VNA", Default {
                                n85 = call "VNA Driver.vi"("Drv Refnum"=w483, "VNA Command"=VNA_Command."CALIBRATE", "error in (no error)"=w485, "Parameters to Measure"=w482) -> ("error out"=w481:errorcluster)  [unwired: 3 in, 4 out]
                                }
                                frame "SNA" {
                                n86 = call "SNA Driver.vi"("Drv Refnum"=w487, "SNA Command"=SNA_Command."CALIBRATE", "error in (no error)"=w490, "Parameters to Measure"=w488) -> ("error out"=w486:errorcluster)  [unwired: 3 in, 4 out]
                                }
                                }
                              }
                            }
                            n87 = flat-sequence {
                              tunnel: [w520] -> w424
                              tunnel: w414 -> [w519]
                              tunnel: w420 -> [_]
                              frame #0 {
                                n88 = call "Test Timing Metrics.vi"("Start?"=FALSE, "Timing Metrics In"=w519, "Message"="Driver Calibration Completed: NA") -> ("Timing Metrics Out"=w520:string)  [unwired: 6 out]
                              }
                            }
                            n89 = call "SP Write to INI File.vi"("error in (no error)"=w420, "Requested Stimulus"=w402, "Parameters to Measure"=w401, "Data to Write"=enum16{"Calibration", "Display", "De-Embed"}."Calibration") -> ("error out"=w426:errorcluster)  [unwired: 3 in, 4 out]
                            n90 = Unbundle(w426) -> ("status"=w406:bool)  [unwired: 2 out]
                            n91 = Select(t="ABORT", s=w426, f=w408) -> (s? t:f=w427:string)
                            n92 = Or(x=w405, y=w406) -> (x .or. y?=w407:bool)
                          }
                          frame "Restore" {
                            n93 = case shown="\"SNA\"" w527 {
                              tunnel: w530 -> [w543 w548]
                              tunnel: w523 -> [w542 w547]
                              tunnel: [w541 w546] -> w529
                              tunnel: w528 -> [w540 w545]
                              frame "VNA", Default {
                                n94 = call "VNA Driver.vi"("Drv Refnum"=w540, "VNA Command"=VNA_Command."RESTORE", "error in (no error)"=w543, "Parameters to Measure"=w542) -> ("error out"=w541:errorcluster)  [unwired: 3 in, 4 out]
                              }
                              frame "SNA" {
                                n95 = call "SNA Driver.vi"("Drv Refnum"=w545, "SNA Command"=SNA_Command."RESTORE", "error in (no error)"=w548, "Parameters to Measure"=w547) -> ("error out"=w546:errorcluster)  [unwired: 3 in, 4 out]
                              }
                            }
                            n96 = flat-sequence {
                              tunnel: w532 -> [w550]
                              tunnel: w529 -> [_]
                              tunnel: [w549] -> w531
                              frame #0 {
                                n97 = call "Test Timing Metrics.vi"("Start?"=FALSE, "Timing Metrics In"=w550, "Message"="Driver Calibration Restored: NA") -> ("Timing Metrics Out"=w549:string)  [unwired: 6 out]
                              }
                            }
                            n98 = call "SP Write to INI File.vi"("error in (no error)"=w529, "Requested Stimulus"=w525, "Parameters to Measure"=w524, "Data to Write"=enum16{"Calibration", "Display", "De-Embed"}."Calibration") -> ("error out"=w534:errorcluster)  [unwired: 3 in, 4 out]
                            n99 = Unbundle(w534) -> ("status"=w535:bool)  [unwired: 2 out]
                            n100 = Select(t="ABORT", s=w534, f="") -> (s? t:f=w536:string)
                          }
                          frame "Ignore" {
                            n101 = case shown="\"VNA\", Default" w564 {
                              tunnel: w563 -> [w624 w636]
                              tunnel: w562 -> [w623 w626]
                              tunnel: w553 -> [w615 w630]
                              tunnel: [w618 w631] -> w572
                              tunnel: w571 -> [w620 w629]
                              tunnel: w561 -> [w621 w634]
                              tunnel: [w614 w627] -> w560
                              tunnel: [w613 w625] -> w573
                              frame "VNA", Default {
                                n102 = call "VNA Driver.vi"("Drv Refnum"=w620, "VNA Command"=VNA_Command."SET STIMULUS", "error in (no error)"=w624, "Miscellaneous Parameters"=w623, "VNA Stimulus"=w621, "Parameters to Measure"=w615) -> ("error out"=w616:errorcluster, "dup Drv Refnum"=w619:T6)  [unwired: 1 in, 3 out]
                                n103 = call "VNA Driver.vi"("Drv Refnum"=w619, "VNA Command"=VNA_Command."GET STIMULUS", "error in (no error)"=w616, "Parameters to Measure"=w615) -> ("error out"=w618:errorcluster, "VNA Flat Output"=w613:string, "dup Drv Refnum"=w614:T6)  [unwired: 3 in, 2 out]
                              }
                              frame "SNA" {
                                n104 = call "SNA Driver.vi"("Drv Refnum"=w629, "SNA Command"=SNA_Command."SET STIMULUS", "error in (no error)"=w636, "Miscellaneous Parameters"=w626, "SNA Stimulus"=w634, "Parameters to Measure"=w630) -> ("error out"=w632:errorcluster, "dup Drv Refnum"=w628:T7)  [unwired: 1 in, 3 out]
                                n105 = call "SNA Driver.vi"("Drv Refnum"=w628, "SNA Command"=SNA_Command."GET STIMULUS", "error in (no error)"=w632, "Miscellaneous Parameters"=w626, "Parameters to Measure"=w630) -> ("error out"=w631:errorcluster, "SNA Flat Output"=w625:string, "dup Drv Refnum"=w627:T7)  [unwired: 2 in, 2 out]
                              }
                            }
                            n106 = flat-sequence {
                              tunnel: [w610] -> w569
                              tunnel: w570 -> [w609]
                              tunnel: w572 -> [_]
                              frame #0 {
                                n107 = call "Test Timing Metrics.vi"("Start?"=FALSE, "Timing Metrics In"=w609, "Message"="Driver Stimulus Set and Check Completed: NA") -> ("Timing Metrics Out"=w610:string)  [unwired: 6 out]
                              }
                            }
                            n108 = call "SP Unpack and Check Stimulus.vi"("Flat Stimulus"=w573, "Requested Stimulus In"=w561) -> ("Stimulus Changed?"=w567:bool, "Current Stimulus"=w566:T11, "Requested Stimulus Out"=w565:T11)  [unwired: 1 out]
                            n109 = case shown="False" w567 {
                              tunnel: [w591 w607] -> w568
                              tunnel: w560 -> [w590 _]
                              tunnel: w564 -> [w589 _]
                              tunnel: w572 -> [w587 w607]
                              tunnel: w559 -> [w586 _]
                              tunnel: w566 -> [w584 _]
                              tunnel: w565 -> [w583 w608]
                              tunnel: [w582 w608] -> w555
                              tunnel: [w581 "MEASURE"] -> w558
                              tunnel: w557 -> [w580 w605]
                              tunnel: [w579 w605] -> w556
                              frame True {
                                n110 = call "SP VNA Cannot Support Measurement Warning.vi"("Current Stimulus"=w584, "Requested Stimulus"=w583, "error in (no error)"=w587, "Instrument IDN String (\"\")"=w586) -> ("error out"=w588:errorcluster, "Choice"=w585:T44)  [unwired: 2 in, 4 out]
                                n111 = case shown="\"Abort\"" w585 {
                                tunnel: [w596 w598 w602] -> w591
                                tunnel: w590 -> [_ _ _]
                                tunnel: w589 -> [_ _ _]
                                tunnel: w588 -> [w596 w598 w602]
                                tunnel: w584 -> [w593 _ _]
                                tunnel: w583 -> [_ w600 w604]
                                tunnel: [w593 w600 w604] -> w582
                                tunnel: ["MEASURE" "ABORT" "ABORT ALL"] -> w581
                                tunnel: w580 -> [w594 w597 w601]
                                tunnel: [w592 w597 w601] -> w579
                                frame "Ignore", Default {
                                n112 = Bundle By Name(cluster=w594, "Stimulus"=w593) -> (w592:T10)
                                }
                                frame "Abort" {
                                }
                                frame "Abort All" {
                                }
                                }
                              }
                              frame False {
                              }
                            }
                            n113 = call "SP Write to INI File.vi"("error in (no error)"=w568, "Requested Stimulus"=w555, "Parameters to Measure"=w554, "Data to Write"=enum16{"Calibration", "Display", "De-Embed"}."Calibration") -> ("error out"=w574:errorcluster)  [unwired: 3 in, 4 out]
                            n114 = Select(t="ABORT", s=w574, f=w558) -> (s? t:f=w578:string)
                          }
                          frame "Abort" {
                            n115 = call "SP Clear Calibration From INI File.vi"("error in (no error)"=w642, "Parameters to Measure"=w637) -> ("error out"=w641:errorcluster)  [unwired: 9 out]
                          }
                          frame "Abort All" {
                            n116 = call "SP Clear Calibration From INI File.vi"("error in (no error)"=w650, "Parameters to Measure"=w645) -> ("error out"=w649:errorcluster)  [unwired: 9 out]
                          }
                        }
                      }
                    }
                  }
                }
              }
              n117 = call "Set LabVIEW VI Topmost.vi"("error in (no error)"=w105, "VI Refnum (null)"=w103) -> ("error out"=w104:errorcluster)  [unwired: 7 in, 2 out]
              n118 = for {
                tunnel: [w113] -> w69 mode=indexing
                tunnel: w68 -> [w112] mode=indexing
                shift-right: [w110] -> w65
                shift-left: w62 -> [w109]
                n119 = Unbundle By Name(w112) -> ("Calibration.String"=w111:string, "Calibration.State"=w113:bool)
                n120 = case shown="Default" w111 {
                  selector: w111 -> [w114 _]
                  tunnel: [w114 w115] -> w110
                  tunnel: w109 -> [_ w115]
                  frame Default {
                  }
                  frame "Not Calibrated" {
                  }
                }
              }
              n121 = And Array Elements(Boolean array=w69) -> (logical AND=w63:bool)
              n122 = Select(t=w65, s=w63, f=w62) -> (s? t:f=w64:string)
              n123 = Bundle By Name(cluster=w67, "Stimulus.Calibration.String"=w64, "Stimulus.Calibration.State"=w63) -> (w66:T10)
            }
            frame "Data File" {
              # "Import data using the S2P IMP Driver."
              n124 = flat-sequence {
                tunnel: [w672] -> w658
                tunnel: w656 -> [w673]
                tunnel: w655 -> [_]
                tunnel: w658 -> [w677]
                tunnel: [w676] -> w657
                tunnel: w654 -> [_]
                frame #0 {
                  n125 = call "Test Timing Metrics.vi"("Start?"=FALSE, "Timing Metrics In"=w673, "Message"="Driver Loaded: IMP") -> ("Timing Metrics Out"=w672:string)  [unwired: 6 out]
                }
                frame #1 {
                  n126 = call "Test Timing Metrics.vi"("Start?"=FALSE, "Timing Metrics In"=w677, "Message"="Driver Initialized: IMP") -> ("Timing Metrics Out"=w676:string)  [unwired: 6 out]
                }
              }
              n127 = call "IMP Driver.vi"("IMP Driver (\"\")"="S2P IMP" ("IMP Driver (\"\")"), "IMP Command"=IMP_Command."LOAD", "error in (no error)"=w669) -> ("error out"=w655:errorcluster, "dup Drv Refnum"=w664:T8)  [unwired: 3 in, 4 out]
              n128 = Bundle By Name(cluster=w667, "IMP Driver Ref"=w664) -> (w666:T5)
              n129 = call "IMP Driver.vi"("Drv Refnum"=w664, "IMP Command"=IMP_Command."INITIALIZE") -> ("error out"=w654:errorcluster, "Variant Output"=w663:variant)  [unwired: 3 in, 5 out]
              n130 = Variant To Data(error in=w655, type="", Variant=w663) -> (data=w661:string, error out=w660:errorcluster)
            }
          }
        }
      }
    }
  }
  "error out" <- w12
  "Instrument ID" <- w16
  "dup Test Parameters" <- w9
  "Next Action" <- w14
  "Parameters to Measure" <- w13
  "Driver Ref" <- w8
  "Timing Metrics Out" <- w6
